vi "[FGV] CaliperEntry_Overlay.vi"(6 "CoordSystemRun":bool=TRUE, 7 "Action":T6, 8 "error in (no error)":errorcluster, 11 "CaliperEntriesIn":T1[](array[typedef]) {"CaliperType" items=["Distance", "Mid Point", "Perpendicular Projection", "Lines Intersection", "Angle from Horizontal", "Angle from Vertical", "Angle Defined by 3 Points", "Angle Defined by 4 Points", "Bissecting Line", "Mid Line", "Center of Mass", "Area", "Line Fit", "Circle Fit", "Ellipse Fit"]}) -> (0 "error out":errorcluster, 3 "AllCaliperEntries":T1[](array[typedef]) {"CaliperType" items=["Distance", "Mid Point", "Perpendicular Projection", "Lines Intersection", "Angle from Horizontal", "Angle from Vertical", "Angle Defined by 3 Points", "Angle Defined by 4 Points", "Bissecting Line", "Mid Line", "Center of Mass", "Area", "Line Fit", "Circle Fit", "Ellipse Fit"]})   [LabVIEW 2019]
uses:
  Controls/Caliper_Entry_FGV_Action.ctl
  Controls/CaliperDataEntry.ctl
  Controls/CaliperType.ctl
  Controls/SelectionListEntry.ctl
  Controls/SelectionListEntryPointType.ctl
  Controls/CaliperResult.ctl
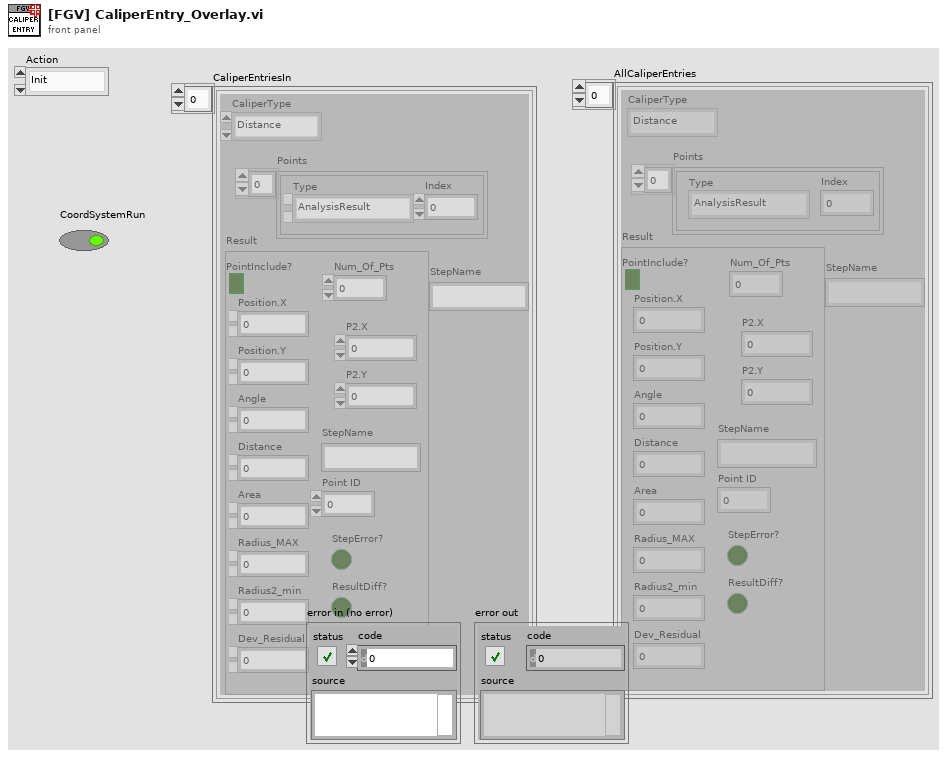
[diagram p1: front panel]
types:
  T1 = typedef "CaliperDataEntry.ctl" = cluster{"CaliperType":T2, "Points":T3[], "Result":T5, "StepName":string}
  T2 = typedef "CaliperType.ctl" = u32
  T3 = typedef "SelectionListEntry.ctl" = cluster{"Type":T4, "Index":i32}
  T4 = typedef "SelectionListEntryPointType.ctl" = enum16{"AnalysisResult", "CaliperResult"}
  T5 = typedef "CaliperResult.ctl" = cluster{"PointInclude?":bool, "Num_Of_Pts":u8, "Position.X":dbl, "Position.Y":dbl, "Angle":dbl, "Distance":dbl, "Area":dbl, "Radius_MAX":dbl, "Radius2_min":dbl, "Dev_Residual":dbl, "P2.X":dbl, "P2.Y":dbl, "StepName":string, "Point ID":u8, "StepError?":bool, "ResultDiff?":bool}
  T6 = typedef "Caliper_Entry_FGV_Action.ctl" = enum16{"Init", "Close", "Add", "Delete", "ReplaceAll", "ReadAll"}
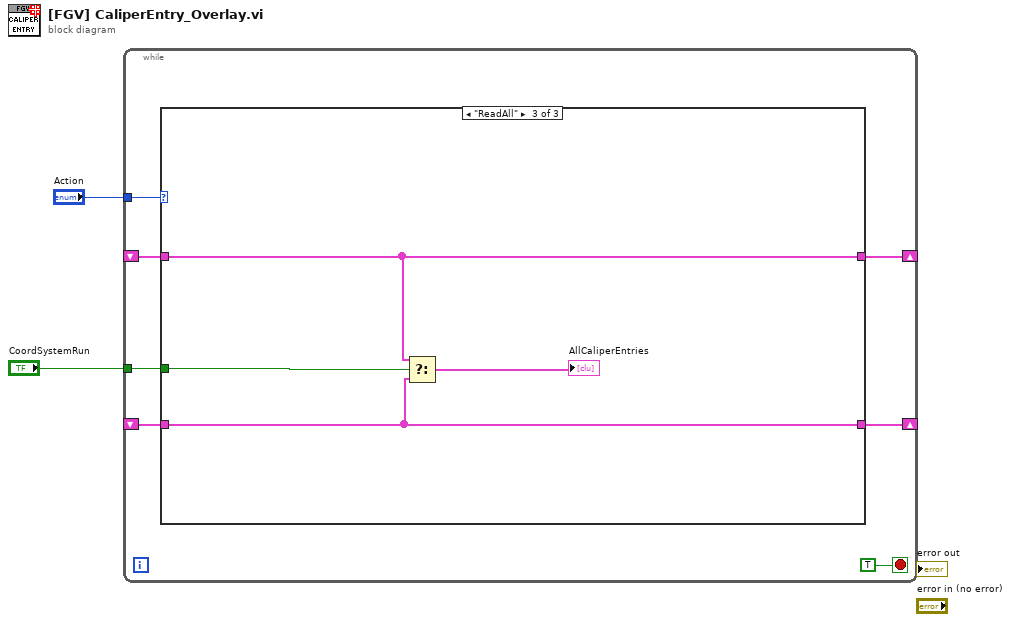
[diagram p0: block diagram]
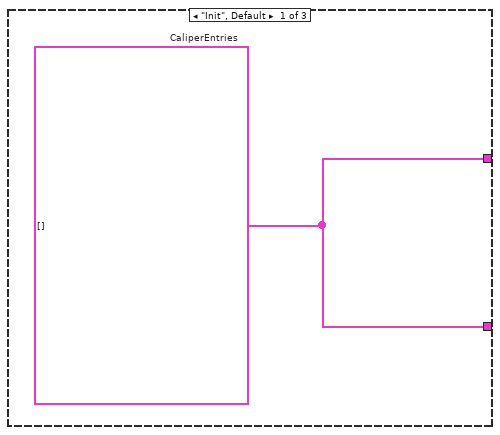
[diagram p2: hidden frame]
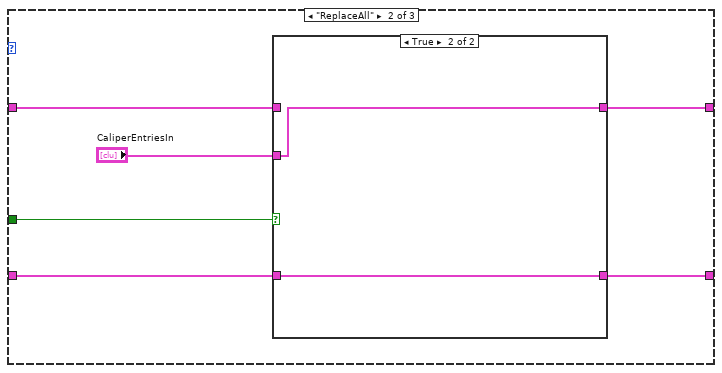
[diagram p3: hidden frame]
diagram:
  n1 = while {
    tunnel: "Action" -> [w8]
    shift-right: [w7] -> _
    shift-left: _ -> [w6]
    tunnel: "CoordSystemRun" -> [w3]
    shift-right: [w5] -> _
    shift-left: _ -> [w4]
    stop <- TRUE stop-if-true
    n2 = case shown="\"ReadAll\"" w8 {
      tunnel: [w10 w14 w23] -> w7
      tunnel: w6 -> [_ w15 w23]
      tunnel: [w10 w11 w21] -> w5
      tunnel: w4 -> [_ w12 w21]
      tunnel: w3 -> [_ w16 w24]
      frame "Init", Default {
        w10 = T1[] []  # CaliperEntries
      }
      frame "ReplaceAll" {
        n3 = case shown="True" w16 {
          tunnel: w15 -> [w18 _]
          tunnel: [w18 w20] -> w14
          tunnel: "CaliperEntriesIn" -> [w17 w20]
          tunnel: w12 -> [_ w19]
          tunnel: [w17 w19] -> w11
          frame False {
          }
          frame True {
          }
        }
      }
      frame "ReadAll" {
        n4 = Select(t=w23, s=w24, f=w21) -> (s? t:f=→"AllCaliperEntries":T1[])
      }
    }
  }
